vi "from string.vi"(8 "error in":errorcluster, 9 "data":string, 10 "version":string, 11 "engine configuration in":refnum<class "base TBM sequencer configuration.lvclass">) -> (0 "error out":errorcluster, 3 "engine configuration out":refnum<class "base TBM sequencer configuration.lvclass">)   [LabVIEW 2014, in "base TBM sequencer configuration.lvclass"]
doc: "Takes a version and data string and unflattens the data back into an Engine Configuration object."
uses:
  base TBM sequencer configuration.lvclass
  Module Mappings.ctl
  <vilib>/NI/Tag Bus/table/mapping specification.ctl
  <vilib>/NI/Tag Bus/tag/Data Type.ctl
  <vilib>/NI/Tag Bus/table/mapping.ctl
  Tag Info.ctl
  <vilib>/NI/Tag Bus Module Framework/channel/TBM channel.lvclass
  base TBM sequencer configuration.lvclass/base TBM sequencer configuration.ctl
  <vilib>/NI/Tag Bus Module Framework/module configuration/TBM module configuration.lvclass
  <vilib>/NI/Tag Bus/tag/tag descriptor.lvclass
  <vilib>/NI/Tag Bus/table/data table.lvlib
  <vilib>/NI/Configuration Framework/serializable configuration/NISE_CEF_serializable configuration.lvclass
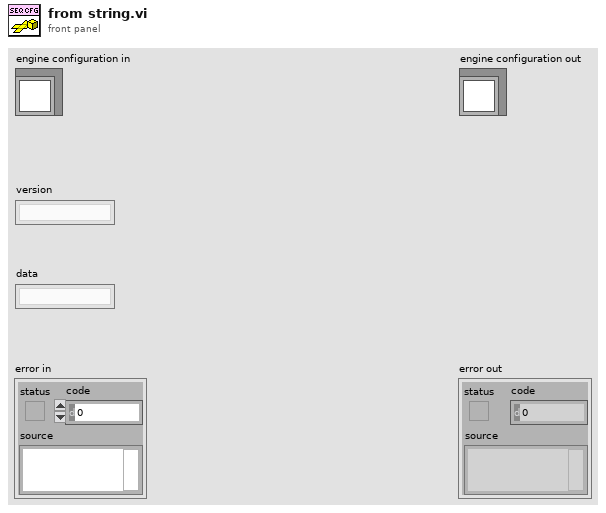
[diagram p1: front panel]
types:
  T1 = typedef "base TBM sequencer configuration.lvclass/Tag Info.ctl" = cluster{"Channel":refnum<class "TBM channel.lvclass">, "Writers":string[], "Readers":string[], "Owning ID":string}
  T2 = typedef "base TBM sequencer configuration.lvclass/Module Mappings.ctl" = cluster{"Owning ID":string, "Input Mappings":T3[], "Process Parameter Mappings":T3[], "Process Results Mappings":T3[], "Output Mappings":T3[]}
  T3 = typedef "tag bus.lvlib/data table.lvlib/mapping specification.ctl" = cluster{"data type":T4, "mappings":T5[]}
  T4 = typedef "tag bus.lvlib/tag descriptor.lvclass/Data Type.ctl" = enum16{"Double", "Single", "I64", "I32", "I16", "I8", "U64", "U32", "U16", "U8", "Boolean", "String", "Array of Double", "Array of Single", "Array of I64", "Array of I32", "Array of I16", "Array of I8", "Array of U64", "Array of U32", "Array of U16", "Array of U8", "Array of Boolean", "Array of String"}
  T5 = typedef "tag bus.lvlib/data table.lvlib/mapping.ctl" = cluster{"sink name":string, "source name":string}
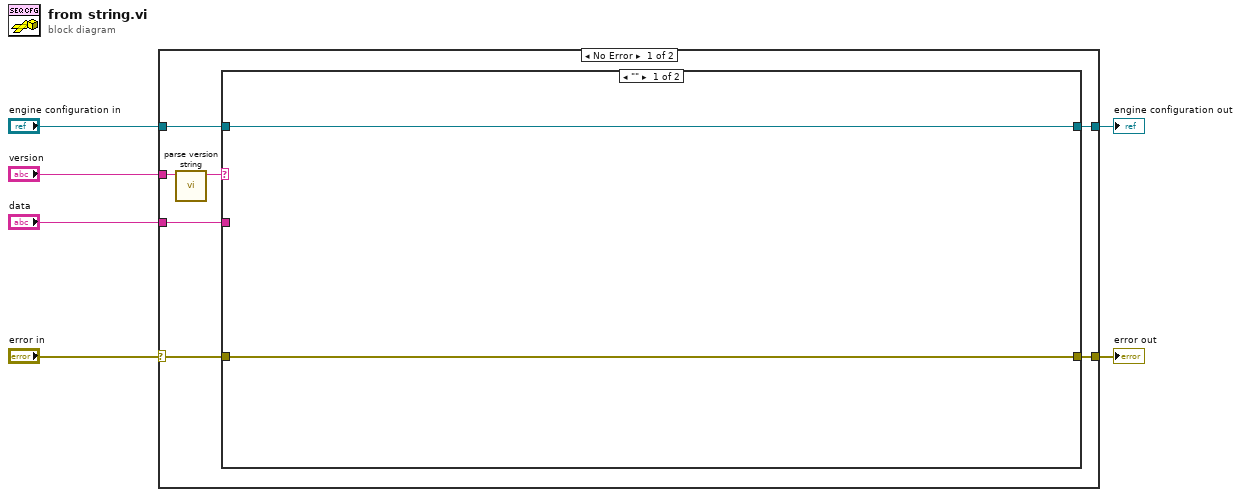
[diagram p0: block diagram]
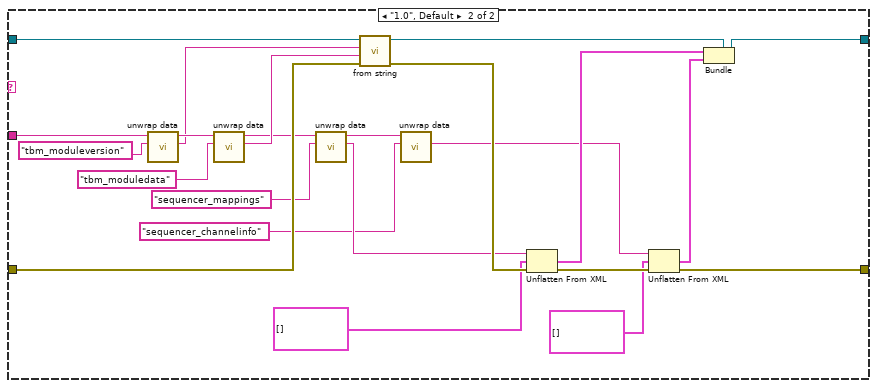
[diagram p2: hidden frame]
diagram:
  n1 = case shown="No Error" "error in" {
    selector: "error in" -> [w9 w40]
    tunnel: "data" -> [w13 _]
    tunnel: "engine configuration in" -> [w12 w39]
    tunnel: [w11 w39] -> w4
    tunnel: [w10 w40] -> w3
    tunnel: "version" -> [w8 _]
    frame No Error {
      n2 = call <vilib>:"parse version string.vi"("full version"=w8) -> ("major.minor version"=w7:string)  [unwired: 7 in, 3 out]
      n3 = case shown="\"\"" w7 {
        tunnel: w9 -> [w14 w38]
        tunnel: w13 -> [_ w32]
        tunnel: w12 -> [w15 w37]
        tunnel: [w15 w28] -> w11
        tunnel: [w14 w27] -> w10
        frame "" {
        }
        frame "1.0", Default {
          n4 = call <vilib>:"unwrap data.vi"("identifier"="tbm_moduleversion" ("additional identifier"), "data to unwrap"=w32) -> ("unwrapped data"=w31:string, "remaining string"=w34:string)  [unwired: 8 in]
          n5 = call <vilib>:"unwrap data.vi"("identifier"="tbm_moduledata" ("additional identifier"), "data to unwrap"=w34) -> ("unwrapped data"=w30:string, "remaining string"=w22:string)  [unwired: 8 in]
          n6 = call <vilib>:"unwrap data.vi"("identifier"="sequencer_mappings" ("additional identifier"), "data to unwrap"=w22) -> ("unwrapped data"=w19:string, "remaining string"=w21:string)  [unwired: 8 in]
          n7 = call-parent "from string.vi"("error in"=w38, "data"=w30, "version"=w31, "module configuration in"=w37) -> ("error out"=w35:errorcluster, "module configuration out"=w36:refnum<class "base TBM sequencer configuration.lvclass">)  [unwired: 6 in]
          n8 = call <vilib>:"unwrap data.vi"("identifier"="sequencer_channelinfo" ("additional identifier"), "data to unwrap"=w21) -> ("unwrapped data"=w20:string)  [unwired: 8 in, 1 out]
          n9 = Unflatten From XML(xml string=w19, type=T1[] [] ("Tag List"), error in (no error)=w35) -> (value=w23:T1[], error out=w29:errorcluster)
          n10 = Unflatten From XML(xml string=w20, type=T2[] [] ("module Mappings"), error in (no error)=w29) -> (value=w25:T2[], error out=w27:errorcluster)
          n11 = Bundle(cluster=w36, w23, w25) -> (w28:refnum<class "base TBM sequencer configuration.lvclass">)
        }
      }
    }
    frame Error {
    }
  }
  "error out" <- w3
  "engine configuration out" <- w4
